vi "Current Read Single.vi"(9 "Channel Index":i32=1, 11 "Device in":refnum<class "Device.lvclass">) -> (1 "Changed or First Call?":bool, 2 "Current.chX.SP":dbl, 3 "Device out":refnum<class "Device.lvclass">)   [LabVIEW 2023, in "Device.lvclass"]
uses:
  Device.lvclass
  Device.lvclass/Device.ctl
  Low Level Capabilities/Current/Current Setpoint/Current Setpoint.lvclass
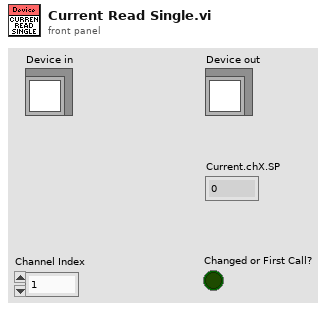
[diagram p1: front panel]
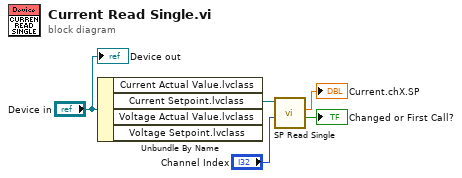
[diagram p0: block diagram]
diagram:
  n1 = Unbundle By Name("Device in") -> ("Current Setpoint.lvclass"=w4:refnum<class "Current Setpoint.lvclass">)  [unwired: 3 out]
  n2 = call-dynamic "SP Read Single.vi"("Channel Index"="Channel Index", "Current Setpoint.lvclass"=w4) -> ("Changed or First Call?"=→"Changed or First Call?":bool, "Current Setpoint"=→"Current.chX.SP":dbl)  [unwired: 6 in, 2 out]
  "Device out" <- "Device in"
